vi "DigitalToString.vi"(9 "D1":bool, 10 "D0":bool) -> (2 "Out":string)   [LabVIEW 2014]
panel:
  out "Led1":bool
  out "Led0":bool
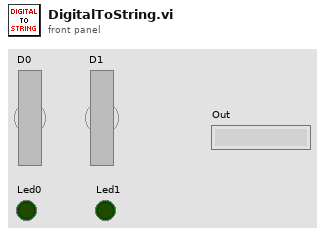
[diagram p1: front panel]
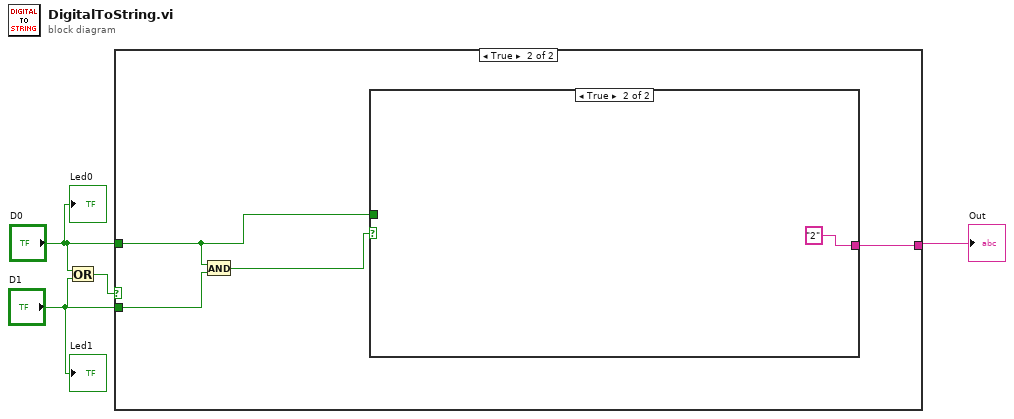
[diagram p0: block diagram]
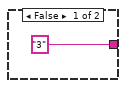
[diagram p2: hidden frame]
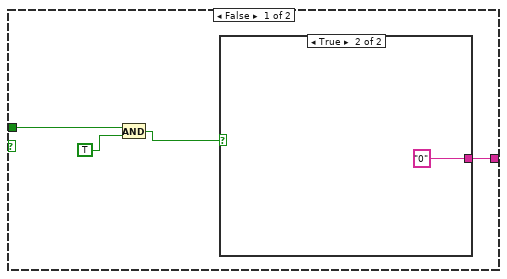
[diagram p3: hidden frame]
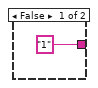
[diagram p4: hidden frame]
diagram:
  n1 = Or(x="D0", y="D1") -> (x .or. y?=w4:bool)
  n2 = case shown="True" w4 {
    tunnel: ["3" w7] -> w3
    tunnel: "D0" -> [_ w6]
    tunnel: "D1" -> [_ w9]
    frame False {
    }
    frame True {
      n3 = And(x=w6, y=w9) -> (x .and. y?=w8:bool)
      n4 = case shown="True" w8 {
        tunnel: [w10 "2"] -> w7
        tunnel: w6 -> [w13 _]
        frame False {
          n5 = And(x=w13, y=TRUE) -> (x .and. y?=w11:bool)
          n6 = case shown="True" w11 {
            tunnel: ["1" "0"] -> w10
            frame False {
            }
            frame True {
            }
          }
        }
        frame True {
        }
      }
    }
  }
  "Out" <- w3
  "Led0" <- "D0"
  "Led1" <- "D1"
